vi "Errors_Global.vi"() -> ()   [LabVIEW 2016]
panel:
  in  "Stop waiting?":bool
  out "Errors":string[](array[string])
  out "Dialog?":bool=TRUE
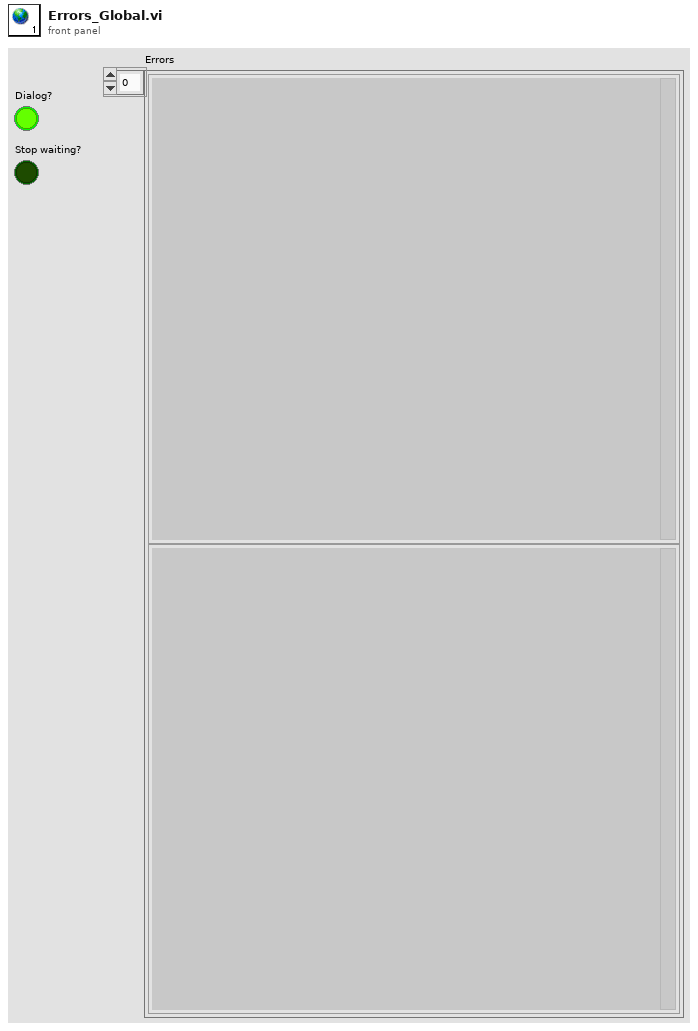
[diagram p1: front panel]
diagram:
